vi "ToZero.vi"(1 "Angle":dbl) -> (0 "Power Change":dbl)   [LabVIEW 2013]
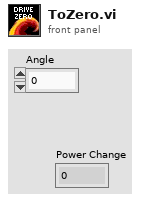
[diagram p1: front panel]
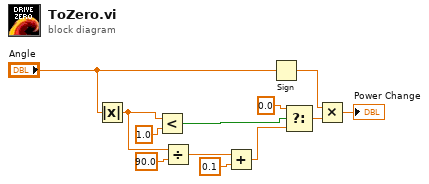
[diagram p0: block diagram]
diagram:
  n1 = Absolute Value(x="Angle") -> (abs(x)=w3:dbl)
  n2 = Less?(x=w3, y=1.0 ("upper limit")) -> (x < y?=w1:bool)
  n3 = Divide(x=w3, y=90.0) -> (x/y=w8:dbl)
  n4 = Add(x=w8, y=0.1) -> (x+y=w9:dbl)
  n5 = Sign(1:"Angle") -> (0:w5:dbl)
  n6 = Select(t=0.0, s=w1, f=w9) -> (s? t:f=w7:dbl)
  n7 = Multiply(x=w5, y=w7) -> (x*y=→"Power Change":dbl)
